vi "decision_path.vi"(8 "error in (no error)":errorcluster caption="entrée d'erreur (pas d'erreur)", 11 "Tree.lvclass":refnum<class "Tree.lvclass">) -> (0 "error out":errorcluster caption="sortie d'erreur", 2 "out":T1, 3 "Tree.lvclass 2":refnum<class "Tree.lvclass">)   [LabVIEW 2020, in "Tree.lvclass"]
doc: "Return the decision path in the tree.\n\n .. versionadded:: 0.18\n\n Parameters\n ----------\n X : {array-like, sparse matrix} of shape (n_samples, n_features)\n The input samples. Internally, it will be converted to\n ``dtype=np.float32`` and if a sparse matrix is provided\n to a sparse ``csr_matrix``.\n\n check_input : bool, default=True\n Allow to bypass several input checking.\n Don't use this parameter unless you know what you do.\n\n Returns\n -------\n indicator : sparse matrix of shape (n_samples, n_nodes)\n Return a node indicator CSR matrix where non zero elements\n indicates that the samples goes through the nodes."
uses:
  Tree.lvclass
  C:/Users/cipop/TDF Dropbox/2_Technologies de France/1 - Services et Etudes/PLAIY/2 - DEV/PLAIYLAB/code/Python/Python.lvclass
  C:/Users/cipop/TDF Dropbox/2_Technologies de France/1 - Services et Etudes/PLAIY/2 - DEV/PLAIYLAB/code/Model/Model.lvclass
  Tree.lvclass/Tree.ctl
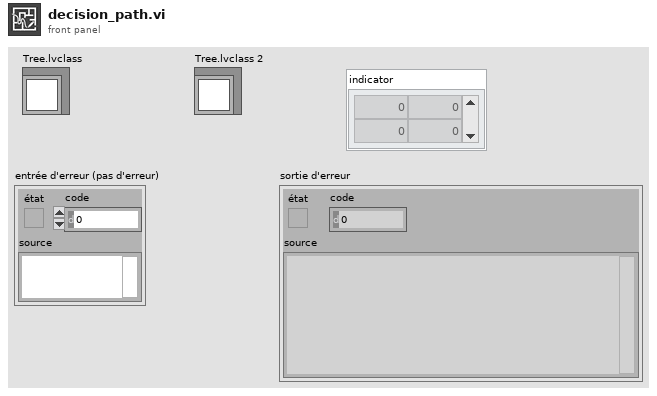
[diagram p1: front panel]
types:
  T1 = cluster{"indicator":dbl[][], "n_nodes_ptr":dbl[]}
  T2 = typedef "data.ctl" = cluster{"name":string, "X":dbl[][]}
  T3 = typedef "tree_data.ctl" = cluster{"y":dbl[][], "sample_weight":dbl[], "check_input":bool}
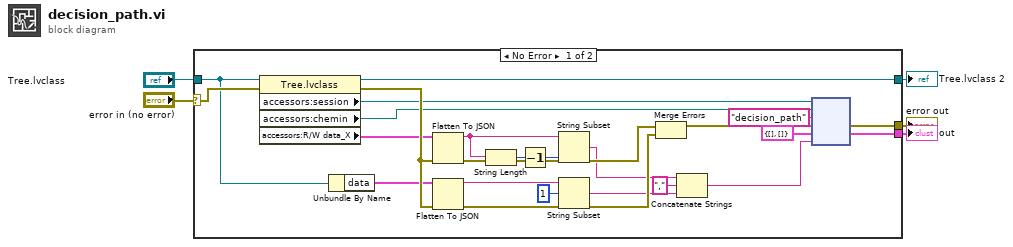
[diagram p0: block diagram]
diagram:
  n1 = case shown="No Error" "error in (no error)" {
    selector: "error in (no error)" -> [w27 w31]
    tunnel: [w28 w31] -> w3
    tunnel: [w10 w30] -> w1
    tunnel: "Tree.lvclass" -> [w9 w30]
    tunnel: [w7 _] -> w5
    frame No Error {
      n2 = property class="Tree.lvclass"(reference=w9, error in=w27) -> (reference out=w10:refnum<class "Tree.lvclass">, error out=w23:errorcluster, "accessors:session"=w13:refnum<k35>, "accessors:chemin"=w12:path, "accessors:R/W data_X"=w14:T2)
      n3 = Unbundle By Name(w9) -> ("data"=w8:T3)
      n4 = Flatten To JSON(anything=w14, error in (no error)=w23) -> (JSON string=w24:string, 11:w19:errorcluster)  [unwired: 1 in]
      n5 = Flatten To JSON(anything=w8, error in (no error)=w23) -> (JSON string=w21:string, 11:w20:errorcluster)  [unwired: 1 in]
      n6 = String Length(string=w24) -> (length=w26:i32)
      n7 = Decrement(x=w26) -> (x-1=w25:i32)
      n8 = String Subset(string=w24, length (rest)=w25) -> (substring=w17:string)  [unwired: 1 in]
      n9 = String Subset(string=w21, offset (0)=1) -> (substring=w16:string)  [unwired: 1 in]
      n10 = Merge Errors(w19, w20) -> (w11:errorcluster)
      n11 = Concatenate Strings(w17, "," ("string"), w16) -> (w15:string)
      n12 = node(w13, w12, "decision_path" ("nom de la fonction"), w11, T1 {"indicator"=[], "n_nodes_ptr"=[]} ("out"), w15) -> (w28:errorcluster, w7:T1)  [unwired: 1 in, 3 out]
    }
    frame Error {
    }
  }
  "out" <- w5
  "error out" <- w3
  "Tree.lvclass 2" <- w1
